vi "Hi-Tec_calibs.vi"(5 "Gas Line Name":string) -> (1 "Hi-Tec calib":T1={"Ref temp (deg C)"=0.0, "Ref Pres (mbars)"=0.0, "Density at calib conditions"=-0.0141, "Coefficients"=[], "Fit"=enum."Cubic Hermite Spline"} {"Coefficients" format="%.2f"; "Density at calib conditions" format="%.4f"; "Ref Pres (mbars)" format="%.2f"; "Ref temp (deg C)" format="%.2f"}, 2 "Comments":string)   [LabVIEW 2022 SP3]
uses:
  Controls/Hi-Tec_calib.ctl
  Controls/Hi-Tec Fitting.ctl
  Anemometry/Anemometry Sub Vis/Globals/Gas_management_global.vi
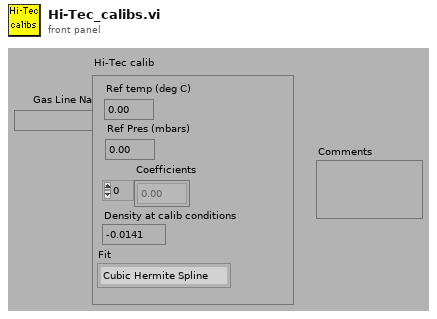
[diagram p1: front panel]
types:
  T1 = typedef "Hi-Tec_calib.ctl" = cluster{"Ref temp (deg C)":dbl, "Ref Pres (mbars)":dbl, "Density at calib conditions":dbl, "Coefficients":dbl[], "Fit":T2}
  T2 = typedef "Hi-Tec Fitting.ctl" = enum16{"Polynomial", "Cubic Hermite Spline"}
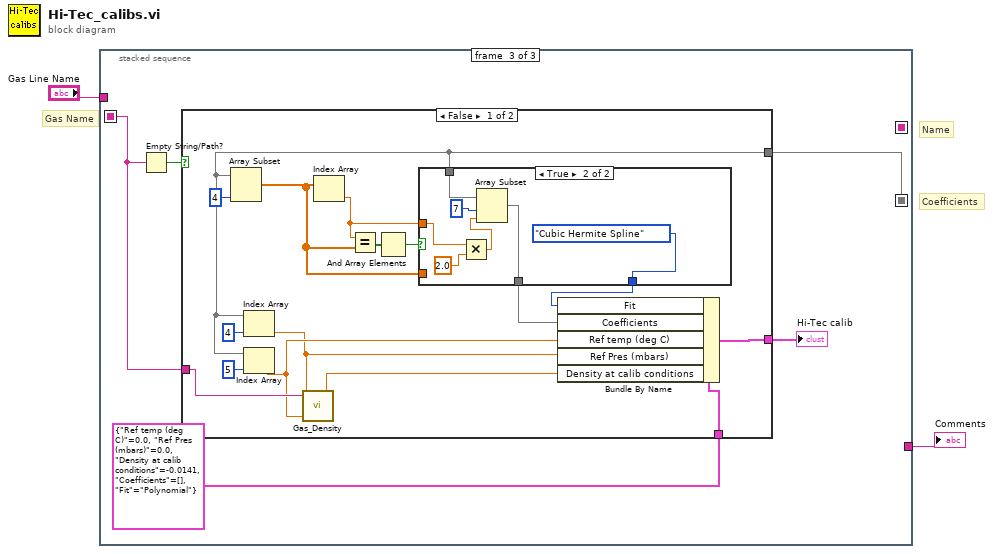
[diagram p0: block diagram]
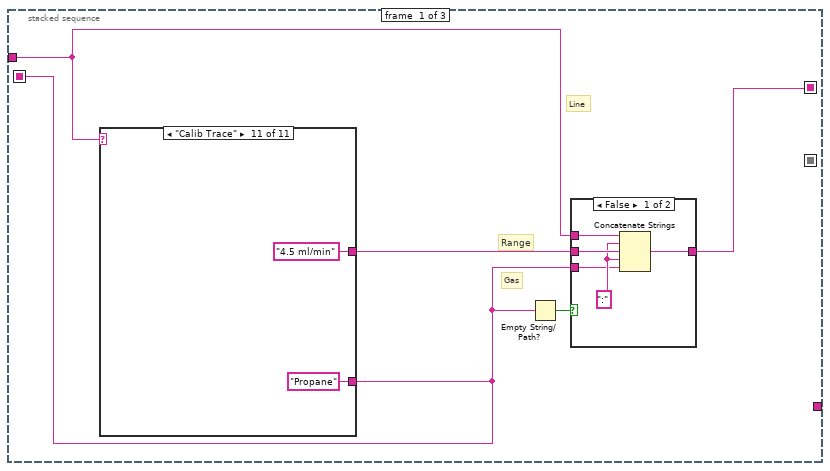
[diagram p2: hidden frame]
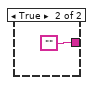
[diagram p3: hidden frame]
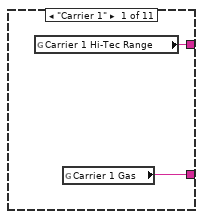
[diagram p4: hidden frame]
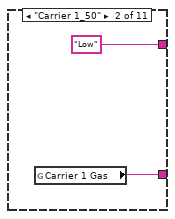
[diagram p5: hidden frame]
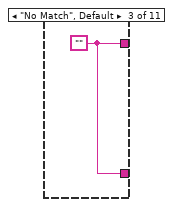
[diagram p6: hidden frame]
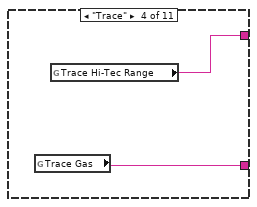
[diagram p7: hidden frame]
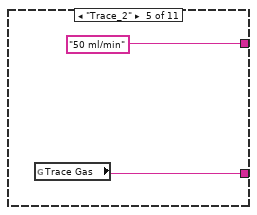
[diagram p8: hidden frame]
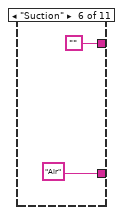
[diagram p9: hidden frame]
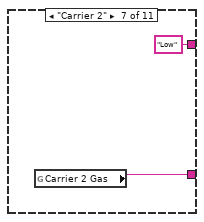
[diagram p10: hidden frame]
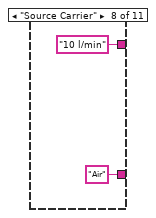
[diagram p11: hidden frame]
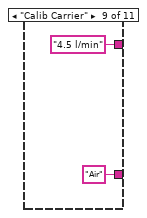
[diagram p12: hidden frame]
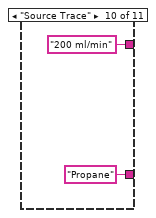
[diagram p13: hidden frame]
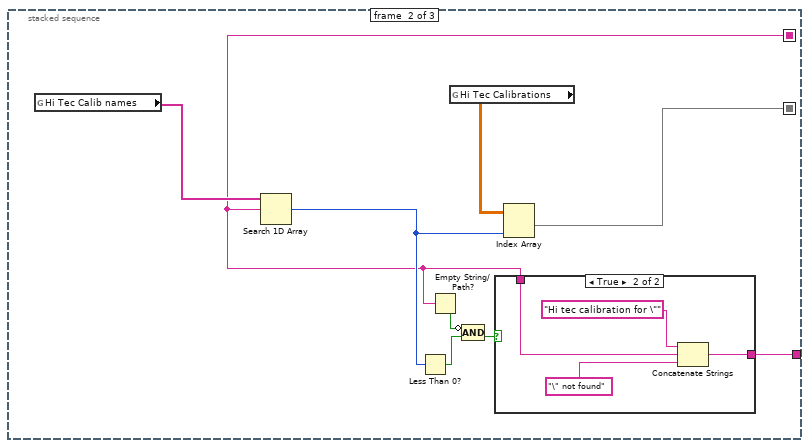
[diagram p14: hidden frame]
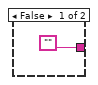
[diagram p15: hidden frame]
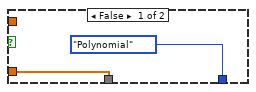
[diagram p16: hidden frame]
diagram:
  # "Name"
  # "Coefficients"
  # "Gas Name"
  n1 = stacked-sequence {
    seq-local: [w5 _ _] -> [_ _ w52]
    seq-local: [_ w41 _] -> [_ _ w49]
    seq-local: [w3 _ _] -> [_ w38 _]
    tunnel: "Gas Line Name" -> [w7 _ _]
    tunnel: [_ w39 _] -> w1
    frame #0 {
      # "Gas"
      # "Range"
      # "Line"
      n2 = case shown="\"Calib Trace\"" w7 {
        tunnel: [w14 "Low" w18 w20 "50 ml/min" ("Trace Hi-Tec Range") "" "Low" "10 l/min" ("Trace Hi-Tec Range") "4.5 l/min" ("Trace Hi-Tec Range") "200 ml/min" ("Trace Hi-Tec Range") "4.5 ml/min" ("Trace Hi-Tec Range")] -> w6
        tunnel: [w15 w17 w18 w19 w22 "Air" ("Carrier 2 Gas") w26 "Air" ("Carrier 2 Gas") "Air" ("Carrier 2 Gas") "Propane" ("Carrier 2 Gas") "Propane" ("Carrier 2 Gas")] -> w5
        frame "Carrier 1" {
          n3 = global read "Gas_management_global.vi" "Carrier 1 Hi-Tec Range"() -> (w14:string)
          n4 = global read "Gas_management_global.vi" "Carrier 1 Gas"() -> (w15:string)
        }
        frame "Carrier 1_50" {
          n5 = global read "Gas_management_global.vi" "Carrier 1 Gas"() -> (w17:string)
        }
        frame "No Match", Default {
          w18 = ""
        }
        frame "Trace" {
          n6 = global read "Gas_management_global.vi" "Trace Gas"() -> (w19:string)
          n7 = global read "Gas_management_global.vi" "Trace Hi-Tec Range"() -> (w20:string)
        }
        frame "Trace_2" {
          n8 = global read "Gas_management_global.vi" "Trace Gas"() -> (w22:string)
        }
        frame "Suction" {
        }
        frame "Carrier 2" {
          n9 = global read "Gas_management_global.vi" "Carrier 2 Gas"() -> (w26:string)
        }
        frame "Source Carrier" {
        }
        frame "Calib Carrier" {
        }
        frame "Source Trace" {
        }
        frame "Calib Trace" {
        }
      }
      n10 = Empty String/Path?(string/path=w5) -> (empty?=w4:bool)
      n11 = case shown="False" w4 {
        tunnel: w7 -> [w12 _]
        tunnel: w6 -> [w11 _]
        tunnel: w5 -> [w9 _]
        tunnel: [w8 ""] -> w3
        frame False {
          w10 = ":"
          n12 = Concatenate Strings(w12, w10, w11, w10, w9) -> (w8:string)
        }
        frame True {
        }
      }
    }
    frame #1 {
      n13 = global read "Gas_management_global.vi" "Hi Tec Calib names"() -> (w43:string[])
      n14 = Search 1D Array(1D array=w43, element=w38) -> (index of element=w40:i32)  [unwired: 1 out]
      n15 = Less Than 0?(x=w40) -> (x < 0?=w36:bool)
      n16 = Empty String/Path?(string/path=w38) -> (empty?=w37:bool)
      n17 = global read "Gas_management_global.vi" "Hi Tec Calibrations"() -> (w42:dbl[][])
      n18 = Compound Arithmetic op=AND(invert w37, w36) -> (w35:bool)
      n19 = case shown="True" w35 {
        tunnel: w38 -> [_ w47]
        tunnel: ["" w45] -> w39
        frame False {
        }
        frame True {
          n20 = Concatenate Strings("Hi tec calibration for \"", w47, "\" not found") -> (w45:string)
        }
      }
      n21 = Index Array(array=w42, index (col)=w40) -> (element=w41:dbl[])  [unwired: 1 in]
    }
    frame #2 {
      n22 = Empty String/Path?(string/path=w52) -> (empty?=w53:bool)
      n23 = case shown="False" w53 {
        tunnel: w52 -> [w68 _]
        tunnel: w49 -> [w56 _]
        tunnel: [w67 w79] -> w51
        tunnel: T1 {"Ref temp (deg C)"=0.0, "Ref Pres (mbars)"=0.0, "Density at calib conditions"=-0.0141, "Coefficients"=[], "Fit"=enum."Polynomial"} ("Hi-Tec calib") -> [w66 w79]
        frame False {
          n24 = Array Subset(array=w56, length=4) -> (w57:dbl[])  [unwired: 1 in]
          n25 = Index Array(array=w56, index=4) -> (element=w61:dbl)
          n26 = Index Array(array=w56, index=5) -> (element=w62:dbl)
          n27 = call "Gas_Density.vi"("Pressure (mbar)"=w62, "Temperature (C)"=w61, "Gas"=w68) -> ("Density (kg/m^3) (= g/l)"=w69:dbl)
          n28 = Index Array(array=w57) -> (element=w55:dbl)  [unwired: 1 in]
          n29 = Equal?(x=w55, y=w57) -> (x = y?=w59:bool[])
          n30 = And Array Elements(Boolean array=w59) -> (logical AND=w60:bool)
          n31 = case shown="True" w60 {
            tunnel: [w71 w76] -> w58
            tunnel: w57 -> [w71 _]
            tunnel: w56 -> [_ w78]
            tunnel: w55 -> [_ w74]
            tunnel: [Hi-Tec_Fitting."Polynomial" ("Fit") Hi-Tec_Fitting."Cubic Hermite Spline" ("Fit")] -> w54
            frame False {
            }
            frame True {
              n32 = Multiply(x=w74, y=2.0) -> (x*y=w72:dbl)
              n33 = Array Subset(array=w78, index=7, length=w72) -> (w76:dbl[])
            }
          }
          n34 = Bundle By Name(cluster=w66, "Fit"=w54, "Coefficients"=w58, "Ref temp (deg C)"=w61, "Ref Pres (mbars)"=w62, "Density at calib conditions"=w69) -> (w67:T1)
        }
        frame True {
        }
      }
      "Hi-Tec calib" <- w51
    }
  }
  "Comments" <- w1
